vi "Relay.vi"   [LabVIEW 2020, in "NI_AdvCtrl_nonlinear.lvlib"]
doc: "LabVIEW no longer supports this VI. You can obtain similar functionality by installing the LabVIEW Simulation Module.\n\nSwitches between two constants. When the relay is on, it remains on until input drops below the value of switch off point. When the relay is off, it remains off until input exceeds the value of switch on point. The relay is predefined in the on state."
uses:
  <vilib>/addons/control/advanced/NI_AdvCtrl_nonlinear.lvlib
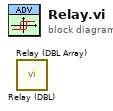
[diagram p0: block diagram]
diagram:
  n1 = call <vilib>:"Relay (DBL).vi"() -> ()  [unwired: 5 in, 1 out]
  n2 = call <vilib>:"Relay (DBL Array).vi"() -> ()  [unwired: 5 in, 1 out]
